vi "3.1.1-VectorNav Read Write.vi"() -> ()   [LabVIEW 2010]
uses:
  3.1.1-VectorNav Registers.ctl
  <vilib>/userDefined/High Color/nirio_resource_hc.ctl
  <vilib>/rvi/interface/nirviOpenFPGA/nirviOpenFPGA.xnode
  2-Low Neurons/2-FPGA VI Typedef.ctl
  FPGA Bitfiles/DaveBrain_FPGATarget_1-Hindbrain_F0E489D8.lvbitx
  1-Hindbrain.vi
  <vilib>/rvi/ClientSDK/nirviWhatTheDeviceIsDoing.ctl
  <vilib>/rvi/interface/nirviCloseFPGA/nirviCloseFPGA.xnode
  <vilib>/FPGAPlugInAG/cRIO-9104/niLvFpga_Open_cRIO-9104.vi
  <vilib>/FPGAPlugInAG/cRIO-9104/niLvFpga_Close_cRIO-9104.vi
panel:
  out "Data":dbl[](array[numeric])
  in  "Command type":T1(ring)
  out "Register":T2
  out "Header":string
  out "error out":errorcluster
  out "Reading":bool=TRUE
  out "Waiting":bool=TRUE
  out "Writing":bool=TRUE
  out "Reply":string
  in  "Manual command":string="$VNRRG,08*7B"
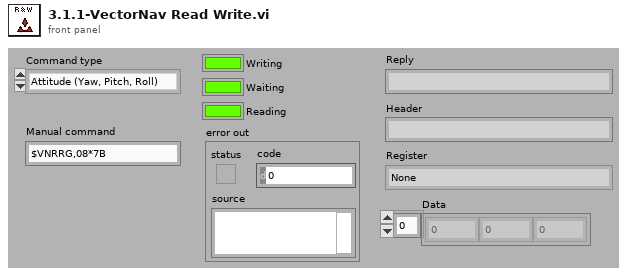
[diagram p1: front panel]
types:
  T1 = enum16{"Attitude (Yaw, Pitch, Roll)", "Tare", "Manual"}
  T2 = typedef "3.1.1-VectorNav Registers.ctl" = enum16{"None", "Model Number", "Hardware Revision", "Serial Number", "Firmware Version", "Serial Baud Rate", "Async Data Output Type", "Async Data Output Freq", "Attitude (Yaw, Pitch, Roll)", "Attitude (Quaternion)"}
  T3 = typedef "nirviWhatTheDeviceIsDoing.ctl" = enum32{"nothing", "something other than LabVIEW FPGA", "FPGA interface", "interactive", "emulation"}
  T4 = typedef "2-FPGA VI Typedef.ctl" = refnum<k20>
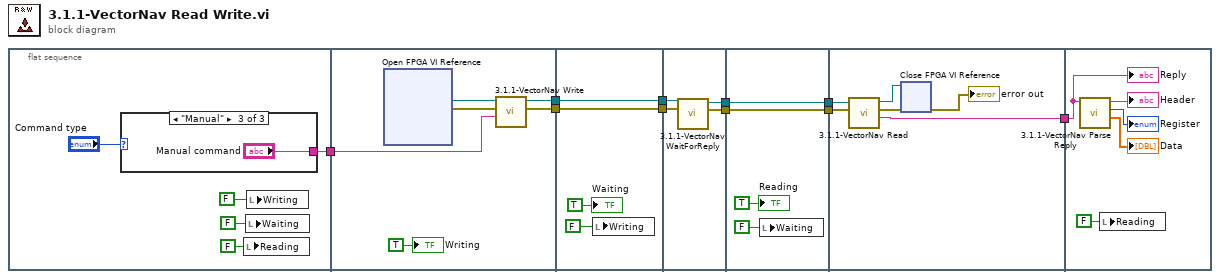
[diagram p0: block diagram]
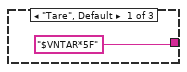
[diagram p2: hidden frame]
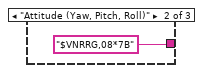
[diagram p3: hidden frame]
diagram:
  n1 = flat-sequence {
    tunnel: [w11] -> w1
    tunnel: [w24] -> w10
    tunnel: [w23] -> w8
    tunnel: w1 -> [w19]
    tunnel: w10 -> [w41]
    tunnel: [w41] -> w9
    tunnel: w8 -> [w40]
    tunnel: [w40] -> w7
    tunnel: w9 -> [w44]
    tunnel: w7 -> [w45]
    tunnel: [w43] -> w6
    tunnel: [w42] -> w4
    tunnel: w6 -> [w49]
    tunnel: [w49] -> w5
    tunnel: w4 -> [w48]
    tunnel: [w48] -> w3
    tunnel: w5 -> [w53]
    tunnel: w3 -> [w52]
    tunnel: [w50] -> w2
    tunnel: w2 -> [w63]
    frame #0 {
      n2 = case shown="\"Manual\"" "Command type" {
        tunnel: ["$VNTAR*5F" "$VNRRG,08*7B" "Manual command"] -> w11
        frame "Tare", Default {
        }
        frame "Attitude (Yaw, Pitch, Roll)" {
        }
        frame "Manual" {
        }
      }
      n3 = local write "Reading"(FALSE ("Writing")) -> ()
      n4 = local write "Waiting"(FALSE ("Writing")) -> ()
      n5 = local write "Writing"(FALSE ("Writing")) -> ()
    }
    frame #1 {
      n6 = xnode "Open FPGA VI Reference"() -> ("FPGA VI Reference Out"=w22:T4, "error out"=w21:errorcluster)  [unwired: 2 in]
      n7 = call "3.1.1-VectorNav Write.vi"("Command"=w19, "error in"=w21, "FPGA VI Reference Out"=w22) -> ("error out"=w23:errorcluster, "FPGA VI Reference Out"=w24:T4)  [unwired: 7 in]
      "Writing" <- TRUE
    }
    frame #2 {
      n8 = local write "Writing"(FALSE ("Writing")) -> ()
      "Waiting" <- TRUE
    }
    frame #3 {
      n9 = call "3.1.1-VectorNav WaitForReply.vi"("error in"=w45, "FPGA VI Reference In"=w44) -> ("error out"=w43:errorcluster, "FPGA VI Reference Out"=w42:T4)  [unwired: 8 in]
    }
    frame #4 {
      n10 = local write "Waiting"(FALSE ("Writing")) -> ()
      "Reading" <- TRUE
    }
    frame #5 {
      n11 = call "3.1.1-VectorNav Read.vi"("error in"=w53, "FPGA VI Reference In"=w52) -> ("Reply"=w50:string, "error out"=w54:errorcluster, "FPGA VI Reference Out"=w55:T4)  [unwired: 7 in]
      n12 = xnode "Close FPGA VI Reference"("FPGA VI Reference In"=w55, "error in"=w54) -> ("error out"=→"error out":errorcluster)
    }
    frame #6 {
      n13 = call "3.1.1-VectorNav Parse Reply.vi"("Input String"=w63) -> ("Data"=→"Data":dbl[], "Register"=→"Register":T2, "Header"=→"Header":string)  [unwired: 8 in]
      n14 = local write "Reading"(FALSE ("Writing")) -> ()
      "Reply" <- w63
    }
  }
